vi "Build Scaled Parameter Data.vi"(8 "error in (no error)":errorcluster, 10 "FPGA Data":u16[](array[numeric]), 11 "Async Message in":refnum<class "Async Message.lvclass">) -> (0 "error out":errorcluster, 1 "Parameter Scaling":T1[](array[typedef]), 2 "Parameter Raw Data":u64[](array[numeric]), 3 "Async Message out":refnum<class "Async Message.lvclass">, 5 "Parameters":string[](array[string]))   [LabVIEW 2020, in "BCI-1553 API.lvlib" / "Async Message.lvclass"]
doc: "<DO NOT CALL>\nRetrieves all the data necessary for the bus controller to perform the scaling operation with protected parent-level VIs."
uses:
  Async Message.lvclass
  TypeDefs/Scaling Information.ctl
  Async Message.lvclass/Async Message.ctl
  BCI-1553 API.lvlib
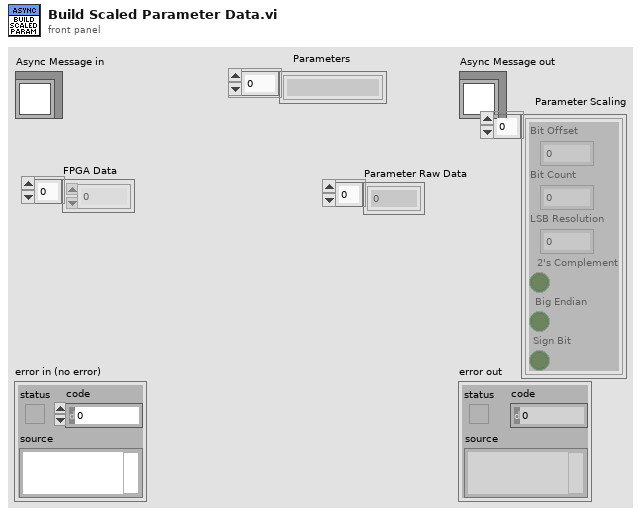
[diagram p1: front panel]
types:
  T1 = typedef "BCI-1553 API.lvlib/Scaling Information.ctl" = cluster{"Bit Offset":i32, "Bit Count":i32, "LSB Resolution":dbl, "2's Complement":bool, "Big Endian":bool, "Sign Bit":bool}
  T2 = typedef "BCI-1553 API.lvlib/Parameter Table Data.ctl" = cluster{"Parameter Name":string, "Base Word":u16, "Address":u16, "Value":u64, "Mask":u16[], "Scaling Info":T1}
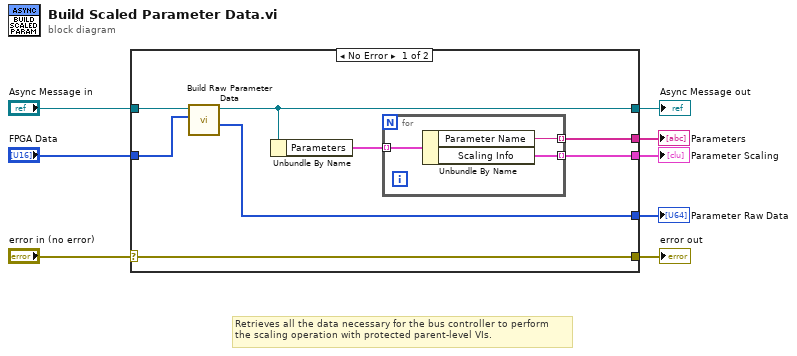
[diagram p0: block diagram]
diagram:
  # "Retrieves all the data necessary for the bus controller to perform\nthe scaling operation with protected parent-level VIs."
  n1 = case shown="No Error" "error in (no error)" {
    selector: "error in (no error)" -> [w16 w21]
    tunnel: [w16 w21] -> w7
    tunnel: [w13 w20] -> w5
    tunnel: "Async Message in" -> [w15 w20]
    tunnel: "FPGA Data" -> [w14 _]
    tunnel: [w11 _] -> w3
    tunnel: [w10 _] -> w1
    tunnel: [w9 _] -> w2
    frame No Error {
      n2 = call-dynamic "Build Raw Parameter Data.vi"("FPGA Data"=w14, "Async Message in"=w15) -> ("Parameter Data"=w9:u64[], "Async Message out"=w13:refnum<class "Async Message.lvclass">)  [unwired: 6 in, 2 out]
      n3 = Unbundle By Name(w13) -> ("Parameters"=w12:T2[])
      n4 = for {
        tunnel: w12 -> [w19] mode=indexing
        tunnel: [w18] -> w11 mode=indexing
        tunnel: [w17] -> w10 mode=indexing
        n5 = Unbundle By Name(w19) -> ("Parameter Name"=w18:string, "Scaling Info"=w17:T1)
      }
    }
    frame Error {
    }
  }
  "error out" <- w7
  "Async Message out" <- w5
  "Parameters" <- w3
  "Parameter Raw Data" <- w2
  "Parameter Scaling" <- w1
